vi "remove duplicate classes.vi"(8 "error in":errorcluster, 9 "class paths in":path[](array[path]), 10 "class names in":string[](array[string]), 11 "discovered classes":path[](array[path])) -> (0 "error out":errorcluster, 1 "class paths out":path[](array[path]), 2 "class names out":string[](array[string]))   [LabVIEW 2013, in "NISE Tools Class Discovery.lvlib"]
doc: "Uses the filename of class files to generate a list of classes and their paths with no duplicates"
uses:
  NISE Tools Class Discovery.lvlib
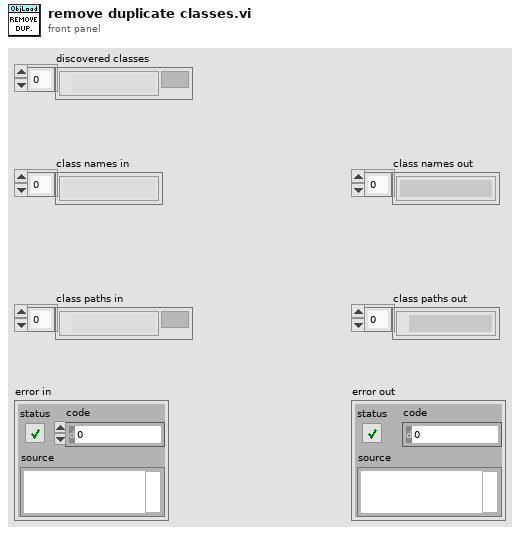
[diagram p1: front panel]
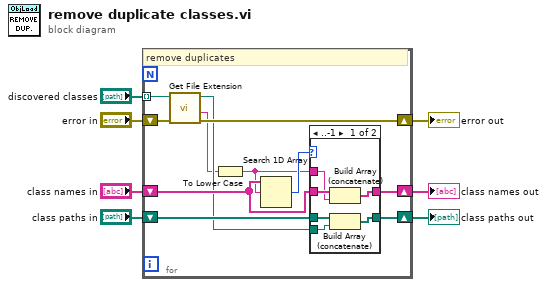
[diagram p0: block diagram]
diagram:
  n1 = for {
    tunnel: "discovered classes" -> [w17] mode=indexing
    shift-right: [w16] -> w7
    shift-left: "error in" -> [w18]
    shift-right: [w12] -> w6
    shift-left: "class names in" -> [w14]
    shift-right: [w11] -> w5
    shift-left: "class paths in" -> [w13]
    # "remove duplicates"
    n2 = call <vilib>:"Get File Extension.vi"("error in (no error)"=w18, "file"=w17) -> ("error out"=w16:errorcluster, "filename without extension"=w9:string, "dup file"=w10:path)  [unwired: 6 in, 1 out]
    n3 = To Lower Case(string=w9) -> (all lower case string=w8:string)
    n4 = Search 1D Array(1D array=w14, element=w8) -> (index of element=w15:i32)  [unwired: 1 in]
    n5 = case shown="..-1" w15 {
      tunnel: w14 -> [w22 w26]
      tunnel: w13 -> [w24 w25]
      tunnel: [w21 w26] -> w12
      tunnel: [w23 w25] -> w11
      tunnel: w10 -> [w20 _]
      tunnel: w8 -> [w19 _]
      frame ..-1 {
        n6 = Build Array (concatenate)(w22, w19) -> (w21:string[])
        n7 = Build Array (concatenate)(w24, w20) -> (w23:path[])
      }
      frame 0.. {
        # "dup"
      }
    }
  }
  "error out" <- w7
  "class names out" <- w6
  "class paths out" <- w5
